vi "Keithley_Standalone_GPIB.vi"() -> ()   [LabVIEW 2018]
uses:
  subVIs/Current_Range_Control.ctl
  <vilib>/Utility/file.llb/Write Delimited Spreadsheet (DBL).vi
panel:
  out "Mean (Ch1/Ch2)":dbl
  out "Ch1/Ch2":dbl
  in  "Time Scale (all t, last f)":bool
  in  "last x seconds":dbl=30.0
  in  "Reset Button":bool
  out "Scan Number":i32
  in  "Current Range Ch 2":T1 items=["Autorange", "+/- 20 mikroA", "+/- 2 mikroA", "+/- 200 nA", "+/- 20 nA", "+/- 2 nA"]
  in  "Current Range Ch 1":T1 items=["Autorange", "+/- 20 mikroA", "+/- 2 mikroA", "+/- 200 nA", "+/- 20 nA", "+/- 2 nA"]
  in  "1D Array Order":i32[](array[numeric])=[1, 4, 3, 6, 2, 5]
  out "Standard Error":dbl[](array[numeric])
  in  "Invert Ch 2":bool
  in  "Invert Ch 1":bool
  out "Chart 2":cluster{"Time Array OUT":dbl[], dbl[]}(graph)
  out "dumped data (%)":dbl
  out "dumped data":i32
  out "t_loop (ms)":u32
  out "use data":bool
  out "error out":errorcluster
  in  "error in (no error)":errorcluster
  in  "GPIB Addr in":refnum<visa-resource-name>="GPIB0::25::INSTR"
  out "Status":i32 format="%.0b"
  out "buffer":string
  out "Chart 1":cluster{"Time Array OUT":dbl[], dbl[]}(graph)
  in  "Stop Keithley":bool
  in  "Sample Rate (Hz) (20)":u32=15
  out "Mean Keithley":dbl[](array[numeric]) format="%#_6e"
  out "SD Keithley":dbl[](array[numeric])
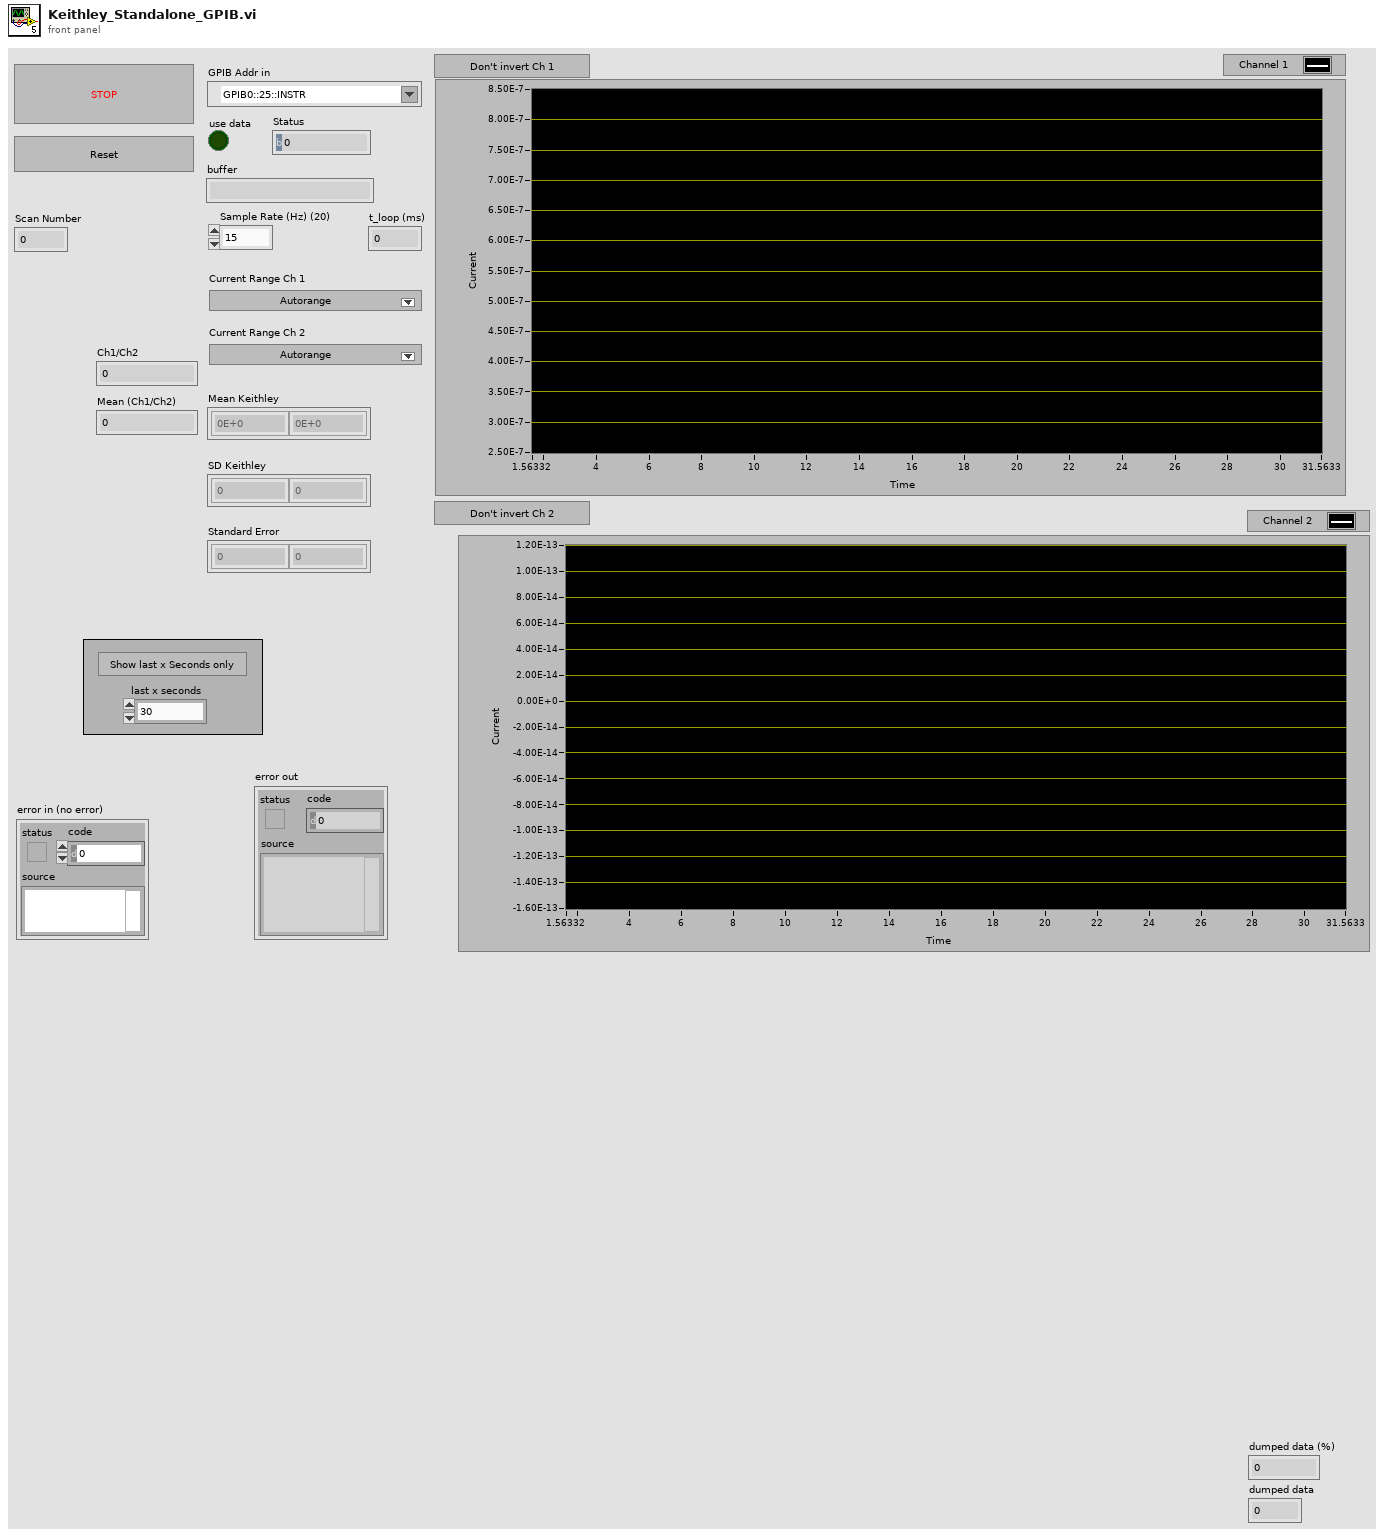
[diagram p1: front panel]
types:
  T1 = typedef "Current_Range_Control.ctl" = u16
  T2 = cluster{"Time Array OUT":dbl[], "Array OUT":dbl[]}
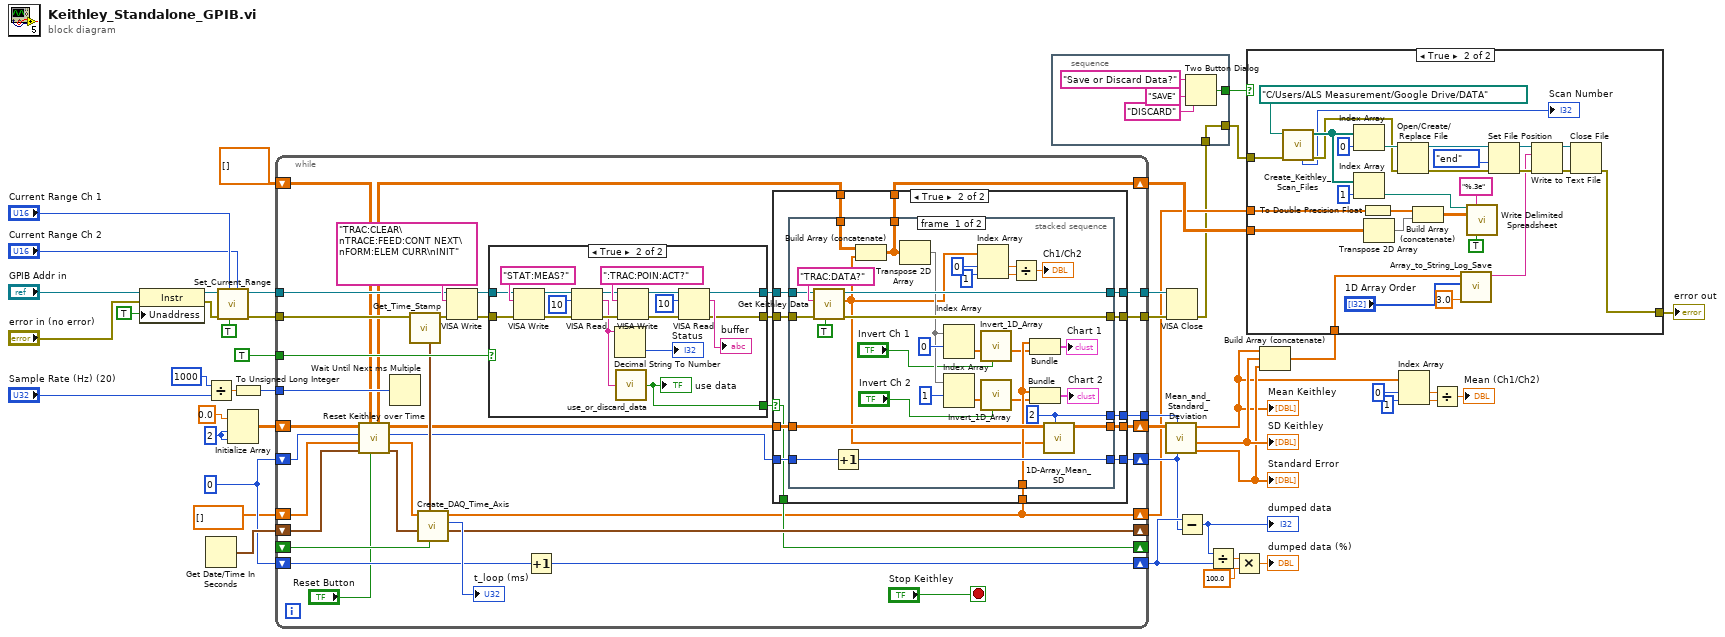
[diagram p0: block diagram]
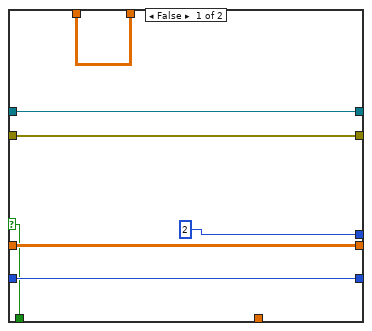
[diagram p3: hidden frame]
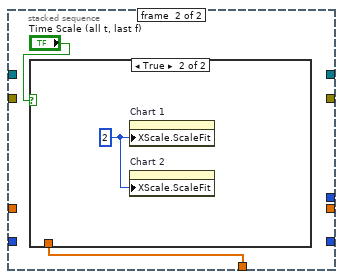
[diagram p4: hidden frame]
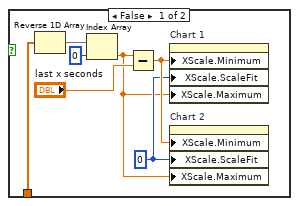
[diagram p5: hidden frame]
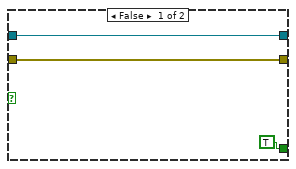
[diagram p6: hidden frame]
diagram:
  w32 = 0
  w44 = 2 ("dimension size")
  n1 = property class="Instr"(reference="GPIB Addr in", error in="error in (no error)", "Unaddress"=TRUE ("GPIB Settings:Unaddressing")) -> (reference out=w23:refnum<visa-resource-name>, error out=w22:errorcluster)
  n2 = Divide(x=1000, y="Sample Rate (Hz) (20)") -> (x/y=w38:dbl)
  n3 = Get Date/Time In Seconds() -> (seconds since 1Jan1904=w35:timestamp)
  n4 = call "Set_Current_Range.vi"("Current Range Ch 2"="Current Range Ch 2", "GPIB (t) / RS-232 (f)"=TRUE, "Current Range Ch 1"="Current Range Ch 1", "error in (no error)"=w22, "VISA resource name"=w23) -> ("error out"=w24:errorcluster, "VISA resource name out"=w25:refnum<visa-resource-name>)  [unwired: 5 in]
  n5 = Initialize Array(0.0 ("element"), w44, w44) -> (w43:dbl[][])
  n6 = To Unsigned Long Integer(number=w38) -> (unsigned 32bit integer=w37:u32)
  n7 = while {
    tunnel: w25 -> [w83]
    tunnel: w24 -> [w67]
    tunnel: [w82] -> w20
    tunnel: [w81] -> w19
    tunnel: TRUE ("Check Completeness of Data (true)") -> [w79]
    shift-right: [w76] -> w41
    shift-left: w43 -> [w58]
    tunnel: [w75] -> w42
    shift-right: [w74] -> w30
    shift-left: w32 -> [w54]
    tunnel: w37 -> [w73]
    shift-right: [w65] -> _
    shift-left: w35 -> [w50]
    shift-right: [w59] -> w17
    shift-left: dbl[] [] ("Time Array OUT") -> [w52]
    shift-right: [w64] -> _
    shift-left: _ -> [w63]
    shift-right: [w61] -> w31
    shift-left: w32 -> [w62]
    shift-right: [w60] -> w18
    shift-left: dbl[][] [] -> [w56]
    stop <- "Stop Keithley" stop-if-true
    n8 = call "Reset Keithley over Time.vi"("Reset Button"="Reset Button", "Data"=w56, "Time Stamp Iteration"=w50, "Time Array IN"=w52, "Iteration Number"=w54, "Mean and SD"=w58) -> ("Time Stamp Iteration out"=w49:timestamp, "Time Array OUT"=w51:dbl[], "Iteration Number out"=w53:i32, "Mean and SD out"=w57:dbl[][], "Data out"=w55:dbl[][])  [unwired: 1 in]
    n9 = Wait Until Next ms Multiple(millisecond multiple=w73) -> ()  [unwired: 1 out]
    n10 = call "Get_Time_Stamp.vi"("error in"=w67) -> ("error out"=w66:errorcluster, "current time"=w69:timestamp)  [unwired: 9 in]
    n11 = call "Create_DAQ_Time_Axis.vi"("NOT [Last Data Point Dumped?]"=w63, "Time Stamp Current Iteration"=w69, "Time Stamp Last Iteration"=w49, "Time Array IN"=w51) -> ("Time Stamp Current Iteration"=w65:timestamp, "Loop Time (ms)"=→"t_loop (ms)":u32, "Time Array OUT"=w59:dbl[])  [unwired: 5 in]
    n12 = VISA Write(VISA resource name=w83, write buffer="TRAC:CLEAR\nTRACE:FEED:CONT NEXT\nFORM:ELEM CURR\nINIT", error in (no error)=w66) -> (VISA resource name out=w80:refnum<visa-resource-name>, error out=w72:errorcluster)  [unwired: 1 out]
    n13 = case shown="True" w79 {
      tunnel: w80 -> [w148 w162]
      tunnel: w72 -> [w147 w161]
      tunnel: [w148 w155] -> w78
      tunnel: [w147 w154] -> w77
      tunnel: [TRUE ("use data") w149] -> w70
      frame False {
      }
      frame True {
        n14 = VISA Write(VISA resource name=w162, write buffer="STAT:MEAS?", error in (no error)=w161) -> (VISA resource name out=w164:refnum<visa-resource-name>, error out=w163:errorcluster)  [unwired: 1 out]
        n15 = VISA Read(VISA resource name=w164, byte count=u32 10, error in (no error)=w163) -> (VISA resource name out=w153:refnum<visa-resource-name>, read buffer=w151:string, error out=w152:errorcluster)  [unwired: 1 out]
        n16 = Decimal String To Number(string=w151) -> (number=→"Status":i32)  [unwired: 2 in, 1 out]
        n17 = call "use_or_discard_data.vi"("Status"=w151) -> ("use data"=w149:bool)
        "use data" <- w149
        n18 = VISA Write(VISA resource name=w153, write buffer=":TRAC:POIN:ACT?", error in (no error)=w152) -> (VISA resource name out=w157:refnum<visa-resource-name>, error out=w156:errorcluster)  [unwired: 1 out]
        n19 = VISA Read(VISA resource name=w157, byte count=u32 10, error in (no error)=w156) -> (VISA resource name out=w155:refnum<visa-resource-name>, read buffer=→"buffer":string, error out=w154:errorcluster)  [unwired: 1 out]
      }
    }
    n20 = Increment(x=w62) -> (x+1=w61:i32)
    n21 = case shown="True" w70 {
      selector: w70 -> [w86 w95]
      tunnel: [w91 w102] -> w82
      tunnel: [w90 w101] -> w81
      tunnel: w78 -> [w91 w104]
      tunnel: w77 -> [w90 w103]
      tunnel: w57 -> [w89 w100]
      tunnel: [w89 w99] -> w76
      tunnel: [2 ("N") w98] -> w75
      tunnel: w53 -> [w87 w97]
      tunnel: [w87 w96] -> w74
      tunnel: [w86 w95] -> w64
      tunnel: [w85 w93] -> w60
      tunnel: w55 -> [w85 w94]
      tunnel: w59 -> [_ w92]
      frame False {
      }
      frame True {
        n22 = stacked-sequence {
          tunnel: w104 -> [w134 _]
          tunnel: w103 -> [w133 _]
          tunnel: [w132 _] -> w102
          tunnel: [w131 _] -> w101
          tunnel: w100 -> [w130 _]
          tunnel: [w129 _] -> w99
          tunnel: [w128 _] -> w98
          tunnel: w97 -> [w127 _]
          tunnel: [w126 _] -> w96
          tunnel: w94 -> [w124 _]
          tunnel: [w121 _] -> w93
          tunnel: w92 -> [w118 w137]
          frame #0 {
            w128 = 2 ("N")
            n23 = call "Get Keithley Data.vi"("GPIB = true, RS-232 = false"=TRUE, "error in (no error)"=w133, "Command"="TRAC:DATA?", "VISA resource name"=w134) -> ("error out"=w131:errorcluster, "Data"=w110:dbl[], "VISA resource name out"=w132:refnum<visa-resource-name>)  [unwired: 4 in, 1 out]
            n24 = Increment(x=w127) -> (x+1=w126:i32)
            n25 = Build Array (concatenate)(w124, w110) -> (w121:dbl[][])
            n26 = Transpose 2D Array(2D array=w121) -> (transposed array=w120:dbl[][])
            n27 = Index Array(array=w120, index (row)=0 ("index")) -> (element=w116:dbl[])  [unwired: 1 in]
            n28 = Index Array(array=w120, index (row)=1 ("index")) -> (element=w115:dbl[])  [unwired: 1 in]
            n29 = Index Array(array=w110, index #1=0 ("index"), index #2=1 ("index")) -> (element #1=w109:dbl, element #2=w108:dbl)
            n30 = call "Invert_1D_Array.vi"("Invert?"="Invert Ch 1", "Array IN"=w116) -> ("Array OUT"=w112:dbl[])  [unwired: 9 in]
            n31 = call "Invert_1D_Array.vi"("Invert?"="Invert Ch 2", "Array IN"=w115) -> ("Array OUT"=w111:dbl[])  [unwired: 9 in]
            n32 = Divide(x=w109, y=w108) -> (x/y=→"Ch1/Ch2":dbl)
            n33 = Bundle("Time Array OUT"=w118, "Array OUT"=w112) -> (→"Chart 1":T2)  [unwired: 1 in]
            n34 = Bundle("Time Array OUT"=w118, "Array OUT"=w111) -> (→"Chart 2":T2)  [unwired: 1 in]
            n35 = call "1D-Array_Mean_SD.vi"("N"=w128, "Data Array"=w110, "IN"=w130) -> ("OUT"=w129:dbl[][])  [unwired: 8 in]
          }
          frame #1 {
            n36 = case shown="True" "Time Scale (all t, last f)" {
              tunnel: w137 -> [w144 _]
              frame False {
                w139 = u8 0
                n37 = Reverse 1D Array(array=w144) -> (reversed array=w143:dbl[])
                n38 = Index Array(array=w143, index=0) -> (element=w138:dbl)
                n39 = Subtract(x=w138, y="last x seconds") -> (x-y=w140:dbl)
                n40 = property on="Chart 1" class="XYGraph (strict)"("XScale.Minimum"=w140, "XScale.ScaleFit"=w139, "XScale.Maximum"=w138) -> ()  [unwired: 2 in, 2 out]
                n41 = property on="Chart 2" class="XYGraph (strict)"("XScale.Minimum"=w140, "XScale.ScaleFit"=w139, "XScale.Maximum"=w138) -> ()  [unwired: 2 in, 2 out]
              }
              frame True {
                w145 = u8 2 ("X Scale.Scale Fit")
                n42 = property on="Chart 1" class="XYGraph (strict)"("XScale.ScaleFit"=w145) -> ()  [unwired: 2 in, 2 out]
                n43 = property on="Chart 2" class="XYGraph (strict)"("XScale.ScaleFit"=w145) -> ()  [unwired: 2 in, 2 out]
              }
            }
          }
        }
      }
    }
  }
  n44 = call "Mean_and_Standard_Deviation.vi"("Iterations"=w30, "Data Points"=w42, "2D array"=w41) -> ("Standard Error"=w7:dbl[], "Standard Deviation"=w8:dbl[], "Mean"=w1:dbl[])  [unwired: 6 in]
  "Mean Keithley" <- w1
  "SD Keithley" <- w8
  "Standard Error" <- w7
  n45 = VISA Close(VISA resource name=w20, error in (no error)=w19) -> (error out=w10:errorcluster)
  n46 = stacked-sequence {
    tunnel: [w171] -> w11
    tunnel: w10 -> [w167]
    tunnel: [w167] -> w9
    frame #0 {
      n47 = Two Button Dialog(message="Save or Discard Data?", 1:"DISCARD" ("F button name (\"Cancel\")"), 2:"SAVE" ("T button name (\"OK\")")) -> (T button?=w171:bool)
    }
  }
  n48 = Subtract(x=w31, y=w30) -> (x-y=w29:i32)
  "dumped data" <- w29
  n49 = Divide(x=w29, y=w31) -> (x/y=w33:dbl)
  n50 = Multiply(x=w33, y=100.0) -> (x*y=→"dumped data (%)":dbl)
  n51 = Build Array (concatenate)(w1, w8, w7) -> (w12:dbl[])
  n52 = case shown="True" w11 {
    tunnel: w18 -> [_ w193]
    tunnel: w17 -> [_ w192]
    tunnel: w9 -> [w172 w177]
    tunnel: [w172 w173] -> w13
    tunnel: w12 -> [_ w174]
    frame False {
    }
    frame True {
      n53 = call "Create_Keithley_Scan_Files.vi"("error in (no error)"=w177, "base path"=path "C:/Users/ALS Measurement/Google Drive/DATA" ("file path (use dialog)")) -> ("error out"=w183:errorcluster, "Save Files Array"=w189:path[], "Scan Number"=→"Scan Number":i32)  [unwired: 5 in, 2 out]
      n54 = Index Array(array=w189, index=0) -> (element=w187:path)
      n55 = Index Array(array=w189, index=1) -> (element=w188:path)
      n56 = To Double Precision Float(number=w192) -> (double precision float=w194:dbl[])
      n57 = Transpose 2D Array(2D array=w193) -> (transposed array=w197:dbl[][])
      n58 = Open/Create/Replace File(file path (use dialog)=w187, error in=w183) -> (refnum out=w186:refnum<file>, error out=w182:errorcluster)  [unwired: 4 in, 1 out]
      n59 = Build Array (concatenate)(w194, w197) -> (w195:dbl[][])
      n60 = call "Array_to_String_Log_Save.vi"("Precision (6)"=3.0, "1D Array Order"="1D Array Order", "1D Array"=w174) -> ("Save String"=w178:string)  [unwired: 7 in, 1 out]
      n61 = call-poly <vilib>:"Write Delimited Spreadsheet.vi"("file path (dialog if empty)"=w188, "format (%.3f)"="%.3e", "2D data"=w195, "transpose? (no:F)"=TRUE) -> ()  [unwired: 10 in, 2 out]
      n62 = Set File Position(refnum=w186, from (0:start)=enum16{"start", "end", "current"}."end", error in=w182) -> (refnum out=w185:refnum<file>, error out=w181:errorcluster)  [unwired: 1 in]
      n63 = Write to Text File(file (use dialog)=w185, text=w178, error in=w181) -> (refnum out=w184:refnum<file>, error out=w180:errorcluster)  [unwired: 1 in, 1 out]
      n64 = Close File(refnum=w184, error in=w180) -> (error out=w173:errorcluster)  [unwired: 1 out]
    }
  }
  "error out" <- w13
  n65 = Index Array(array=w1, index #1=0 ("index"), index #2=1 ("index")) -> (element #1=w2:dbl, element #2=w3:dbl)
  n66 = Divide(x=w2, y=w3) -> (x/y=→"Mean (Ch1/Ch2)":dbl)
